vi "toptopla.vi"() -> ()   [LabVIEW 2015]
panel:
  in  "x":dbl(slide)=-0.34693877551020413 scale=-1.0..1.0
  in  "toplaust":dbl(slide)=0.0816326530612244 scale=-1.0..1.0
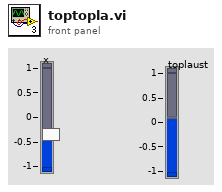
[diagram p1: front panel]
types:
  T1 = typedef "WPI_DigitalInputDevRef.ctl" = cluster{"DevStatus":errorcluster, "DIO Channel":T2}
  T2 = typedef "FPGA_DIOChannel.ctl" = enum8{"DIO 0", "DIO 1", "DIO 2", "DIO 3", "DIO 4", "DIO 5", "DIO 6", "DIO 7", "DIO 8", "DIO 9", "DIO MXP 0", "DIO MXP 1", "DIO MXP 2", "DIO MXP 3", "DIO MXP 4", "DIO MXP 5", "DIO MXP 6", "DIO MXP 7", "DIO MXP 8", "DIO MXP 9", "DIO MXP 10", "DIO MXP 11", "DIO MXP 12", "DIO MXP 13", "DIO MXP 14", "DIO MXP 15", "Invalid"}
  T3 = typedef "WPI_MotorControlDeviceRef.ctl" = cluster{"DeviceStatus":errorcluster, "Type":T4, "PWM":cluster{"PWM Channel":T5, "DeadBand":T6}, "CAN":cluster{"Device Number":u8, "Control Mode":T7, "Semaphore":T8, "Max Vout":dbl, "TalonSRX Control Mode":T9}, "Invert":bool}
  T4 = typedef "WPI_MotorControlType.ctl" = enum16{"PWM", "CAN", "CANTalonSRX"}
  T5 = typedef "FPGA_DIOPWMChannel.ctl" = enum8{"PWM 0", "PWM 1", "PWM 2", "PWM 3", "PWM 4", "PWM 5", "PWM 6", "PWM 7", "PWM 8", "PWM 9", "PWM MXP 0", "PWM MXP 1", "PWM MXP 2", "PWM MXP 3", "PWM MXP 4", "PWM MXP 5", "PWM MXP 6", "PWM MXP 7", "PWM MXP 8", "PWM MXP 9", "Invalid"}
  T6 = typedef "WPI_PWMDeadband.ctl" = cluster{"Name":string, "maxPositivePwm":i32, "minPositivePwm":i32, "centerPwm":i32, "maxNegativePwm":i32, "minNegativePwm":i32, "angularRange":u16}
  T7 = typedef "WPI_CANJaguar_ControlMode.ctl" = enum8{"Percent VBus", "Current", "Speed", "Position", "Voltage"}
  T8 = typedef "Semaphore RefNum" = refnum<k1>
  T9 = typedef "WPI_CANTalonSRX_APIControlMode.ctl" = enum8{"Percent VBus", "Speed", "Position", "Slave", "Unchanged / Invalid", "Voltage Compensation", "Current", "Motion Profile"}
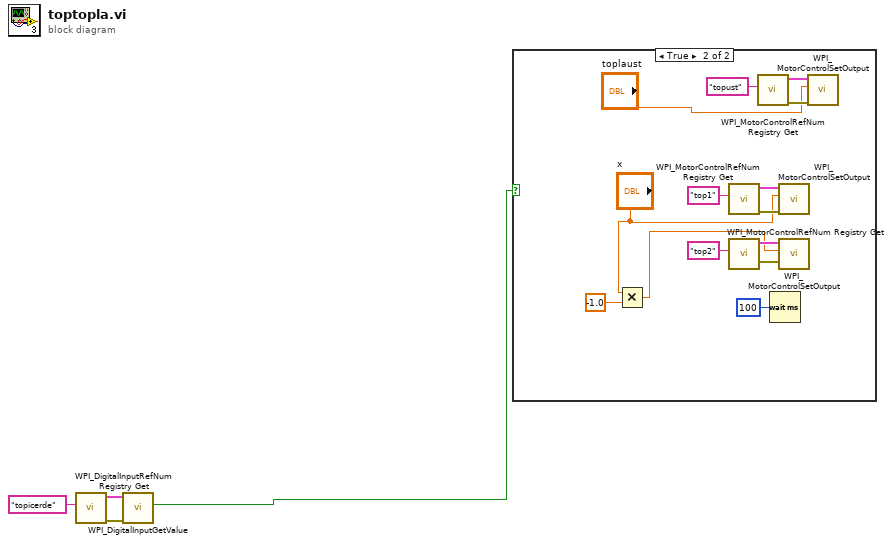
[diagram p0: block diagram]
diagram:
  n1 = call <vilib>:"WPI_DigitalInputRefNum Registry Get.vi"("refnum name"="topicerde") -> ("error out"=w2:errorcluster, "DigitalInputDevRef"=w4:T1)  [unwired: 9 in]
  n2 = call <vilib>:"WPI_DigitalInputGetValue.vi"("error in (no error)"=w2, "DigitalInputDevRef"=w4) -> ("Value"=w1:bool)  [unwired: 7 in, 2 out]
  n3 = case shown="True" w1 {
    frame False {
    }
    frame True {
      n4 = Multiply(x="x", y=-1.0) -> (x*y=w6:dbl)
      n5 = call <vilib>:"WPI_MotorControlRefNum Registry Get.vi"("refnum name"="top1") -> ("error out"=w18:errorcluster, "MotorControlDevRef"=w17:T3)  [unwired: 9 in]
      n6 = call <vilib>:"WPI_MotorControlRefNum Registry Get.vi"("refnum name"="top2") -> ("error out"=w15:errorcluster, "MotorControlDevRef"=w14:T3)  [unwired: 9 in]
      n7 = call <vilib>:"WPI_MotorControlRefNum Registry Get.vi"("refnum name"="topust") -> ("error out"=w12:errorcluster, "MotorControlDevRef"=w11:T3)  [unwired: 9 in]
      n8 = Wait (ms)(milliseconds to wait=u32 100) -> ()  [unwired: 1 out]
      n9 = call <vilib>:"WPI_MotorControlSetOutput.vi"("error in (no error)"=w18, "Output"="x", "MotorControlDevRef"=w17) -> ()  [unwired: 6 in, 3 out]
      n10 = call <vilib>:"WPI_MotorControlSetOutput.vi"("error in (no error)"=w15, "Output"=w6, "MotorControlDevRef"=w14) -> ()  [unwired: 6 in, 3 out]
      n11 = call <vilib>:"WPI_MotorControlSetOutput.vi"("error in (no error)"=w12, "Output"="toplaust", "MotorControlDevRef"=w11) -> ()  [unwired: 6 in, 3 out]
    }
  }
